vi "Untitled 3.vi"(7 "Sheet Name":string, 8 "error in":errorcluster, 9 "Value":bool, 10 "Cell Address":string, 11 "SpreadsheetDocument":refnum<k24>) -> (0 "error out":errorcluster, 3 "SpreadsheetDocument out":refnum<k24>)   [LabVIEW 2025]
uses:
  D:/git/Open-Xml-LabVIEW/dll/DocumentFormat.OpenXml.dll
  dll/DocumentFormat.OpenXml.dll
  Open Xml.lvlib
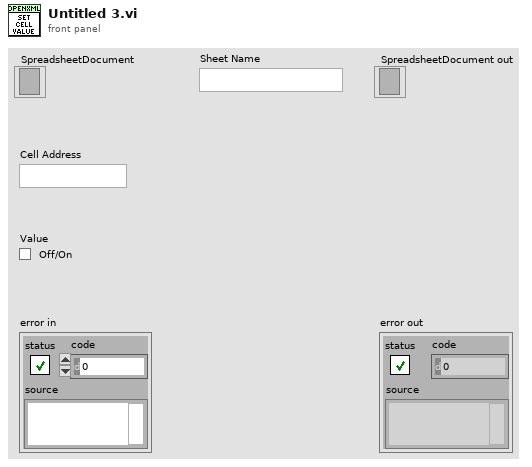
[diagram p1: front panel]
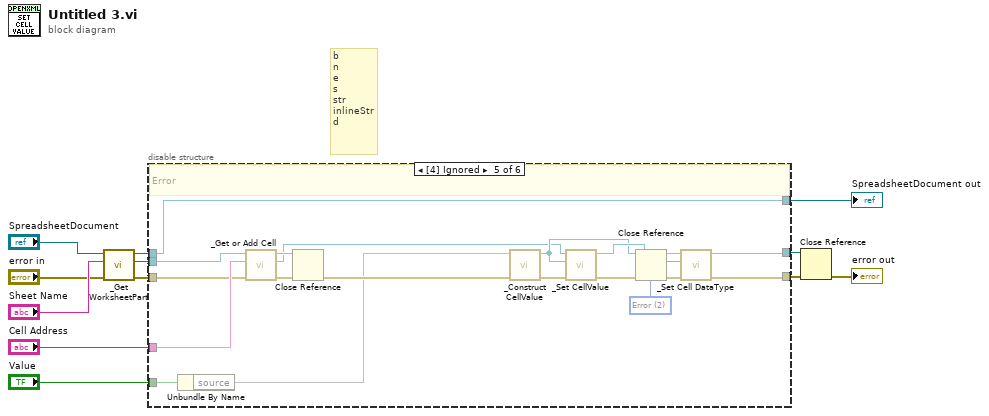
[diagram p0: block diagram]
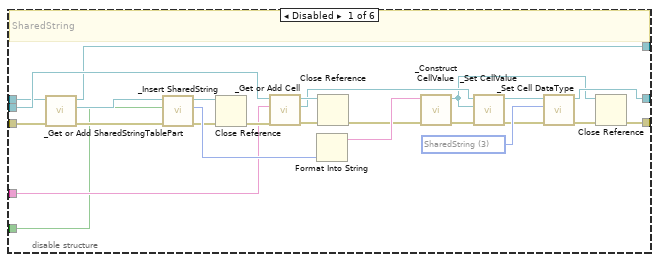
[diagram p2: hidden frame]
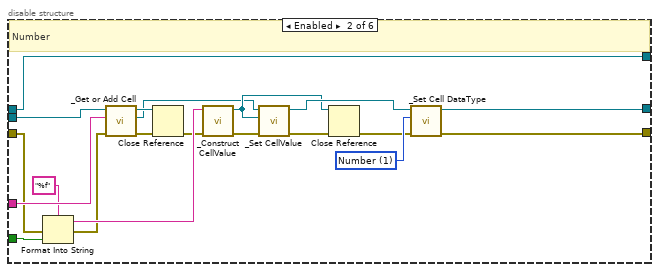
[diagram p3: hidden frame]
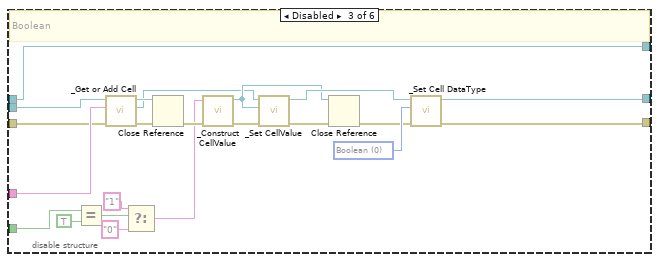
[diagram p4: hidden frame]
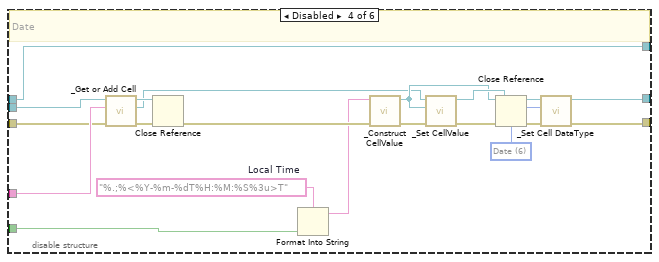
[diagram p5: hidden frame]
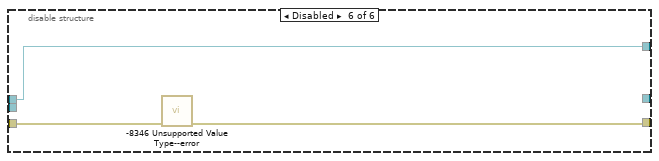
[diagram p6: hidden frame]
diagram:
  # "b\nn\ne\ns\nstr\ninlineStr\nd"
  n1 = call "_Get WorksheetPart.vi"("error in"="error in", "Sheet Name"="Sheet Name", "SpreadsheetDocument in"="SpreadsheetDocument") -> ("error out"=w8:errorcluster, "WorksheetPart"=w7:refnum<k24>, "SpreadsheetDocument out"=w3:refnum<k24>)  [unwired: 6 in]
  n2 = disable-structure shown="[4] Ignored" {
    disable-tunnel: "Value" -> [w17 w53 w64 w81 w100 _]
    disable-tunnel: "Cell Address" -> [w18 w56 w78 w97 w115 _]
    disable-tunnel: w8 -> [w37 w49 w58 w83 w101 w119]
    disable-tunnel: w7 -> [w34 w57 w79 w98 w116 _]
    disable-tunnel: [w14 w47 w74 w93 w111 w117] -> w6
    disable-tunnel: [w28 w46 w73 w92 w110 _] -> w5
    disable-tunnel: w3 -> [w20 w55 w77 w96 w114 w118]
    disable-tunnel: [w19 w55 w77 w96 w114 w118] -> w1
    frame Disabled {
      w16 = 3 items=["Boolean", "Number", "Error", "SharedString", "String", "InlineString", "Date"] ("Datatype")
      # "SharedString"
      n3 = call "_Get or Add SharedStringTablePart.vi"("error in"=w37, "SpreadsheetDoument in"=w20) -> ("error out"=w35:errorcluster, "SharedStringTablePart"=w36:refnum<k24>, "SpreadsheetDocument out"=w19:refnum<k24>)  [unwired: 7 in]
      n4 = call "_Insert SharedString.vi"("error in"=w35, "Value"=w17, "SharedStringTablePart in"=w36) -> ("error out"=w22:errorcluster, "Index"=w25:i32, "SharedStringTablePart out"=w23:refnum<k24>)  [unwired: 6 in]
      n5 = Close Reference(reference=w23, error in (no error)=w22) -> (error out=w24:errorcluster)
      n6 = call "_Get or Add Cell.vi"("error in"=w24, "Cell Address"=w18, "Worksheetpart in"=w34) -> ("error out"=w32:errorcluster, "Cell"=w21:refnum<k24>, "WorksheetPart out"=w26:refnum<k24>)  [unwired: 6 in]
      n7 = Format Into String(w25) -> (resulting string=w33:string)  [unwired: 3 in, 1 out]
      n8 = Close Reference(reference=w26, error in (no error)=w32) -> (error out=w27:errorcluster)
      n9 = call "_Construct CellValue.vi"("error in"=w27, "Text"=w33) -> ("error out"=w31:errorcluster, "CellValue out"=w13:refnum<k24>)  [unwired: 8 in]
      n10 = call "_Set CellValue.vi"("error in"=w31, "CellValue in"=w13, "Cell in"=w21) -> ("error out"=w15:errorcluster, "Cell out"=w30:refnum<k24>)  [unwired: 7 in]
      n11 = call "_Set Cell DataType.vi"("error in"=w15, "Datatype"=w16, "Cell in"=w30) -> ("error out"=w29:errorcluster, "Cell out"=w28:refnum<k24>)  [unwired: 7 in]
      n12 = Close Reference(reference=w13, error in (no error)=w29) -> (error out=w14:errorcluster)
    }
    frame Enabled {
      w43 = 1 items=["Boolean", "Number", "Error", "SharedString", "String", "InlineString", "Date"] ("Datatype")
      # "Number"
      n13 = Format Into String(format string="%f", error in=w49, w53) -> (resulting string=w51:string, error out=w48:errorcluster)  [unwired: 1 in]
      n14 = call "_Get or Add Cell.vi"("error in"=w48, "Cell Address"=w56, "Worksheetpart in"=w57) -> ("error out"=w54:errorcluster, "Cell"=w38:refnum<k24>, "WorksheetPart out"=w39:refnum<k24>)  [unwired: 6 in]
      n15 = Close Reference(reference=w39, error in (no error)=w54) -> (error out=w40:errorcluster)
      n16 = call "_Construct CellValue.vi"("error in"=w40, "Text"=w51) -> ("error out"=w50:errorcluster, "CellValue out"=w41:refnum<k24>)  [unwired: 8 in]
      n17 = call "_Set CellValue.vi"("error in"=w50, "CellValue in"=w41, "Cell in"=w38) -> ("error out"=w44:errorcluster, "Cell out"=w45:refnum<k24>)  [unwired: 7 in]
      n18 = Close Reference(reference=w41, error in (no error)=w44) -> (error out=w42:errorcluster)
      n19 = call "_Set Cell DataType.vi"("error in"=w42, "Datatype"=w43, "Cell in"=w45) -> ("error out"=w47:errorcluster, "Cell out"=w46:refnum<k24>)  [unwired: 7 in]
    }
    frame Disabled {
      w70 = 0 items=["Boolean", "Number", "Error", "SharedString", "String", "InlineString", "Date"] ("Datatype")
      # "Boolean"
      n20 = Equal?(x=w64, y=TRUE) -> (x = y?=w60:bool)
      n21 = call "_Get or Add Cell.vi"("error in"=w58, "Cell Address"=w78, "Worksheetpart in"=w79) -> ("error out"=w76:errorcluster, "Cell"=w65:refnum<k24>, "WorksheetPart out"=w66:refnum<k24>)  [unwired: 6 in]
      n22 = Select(t="1", s=w60, f="0" ("t")) -> (s? t:f=w59:string)
      n23 = Close Reference(reference=w66, error in (no error)=w76) -> (error out=w67:errorcluster)
      n24 = call "_Construct CellValue.vi"("error in"=w67, "Text"=w59) -> ("error out"=w75:errorcluster, "CellValue out"=w68:refnum<k24>)  [unwired: 8 in]
      n25 = call "_Set CellValue.vi"("error in"=w75, "CellValue in"=w68, "Cell in"=w65) -> ("error out"=w71:errorcluster, "Cell out"=w72:refnum<k24>)  [unwired: 7 in]
      n26 = Close Reference(reference=w68, error in (no error)=w71) -> (error out=w69:errorcluster)
      n27 = call "_Set Cell DataType.vi"("error in"=w69, "Datatype"=w70, "Cell in"=w72) -> ("error out"=w74:errorcluster, "Cell out"=w73:refnum<k24>)  [unwired: 7 in]
    }
    frame Disabled {
      w82 = "%.;%<%Y-%m-%dT%H:%M:%S%3u>T"  # Local Time
      w89 = 6 items=["Boolean", "Number", "Error", "SharedString", "String", "InlineString", "Date"] ("Datatype")
      # "Date"
      n28 = call "_Get or Add Cell.vi"("error in"=w83, "Cell Address"=w97, "Worksheetpart in"=w98) -> ("error out"=w95:errorcluster, "Cell"=w84:refnum<k24>, "WorksheetPart out"=w85:refnum<k24>)  [unwired: 6 in]
      n29 = Close Reference(reference=w85, error in (no error)=w95) -> (error out=w86:errorcluster)
      n30 = Format Into String(format string=w82, w81) -> (resulting string=w80:string)  [unwired: 2 in, 1 out]
      n31 = call "_Construct CellValue.vi"("error in"=w86, "Text"=w80) -> ("error out"=w94:errorcluster, "CellValue out"=w87:refnum<k24>)  [unwired: 8 in]
      n32 = call "_Set CellValue.vi"("error in"=w94, "CellValue in"=w87, "Cell in"=w84) -> ("error out"=w90:errorcluster, "Cell out"=w91:refnum<k24>)  [unwired: 7 in]
      n33 = Close Reference(reference=w87, error in (no error)=w90) -> (error out=w88:errorcluster)
      n34 = call "_Set Cell DataType.vi"("error in"=w88, "Datatype"=w89, "Cell in"=w91) -> ("error out"=w93:errorcluster, "Cell out"=w92:refnum<k24>)  [unwired: 7 in]
    }
    frame Disabled {
      w107 = 2 items=["Boolean", "Number", "Error", "SharedString", "String", "InlineString", "Date"] ("Datatype")
      # "Error"
      n35 = Unbundle By Name(w100) -> ("source"=w99)
      n36 = call "_Get or Add Cell.vi"("error in"=w101, "Cell Address"=w115, "Worksheetpart in"=w116) -> ("error out"=w113:errorcluster, "Cell"=w102:refnum<k24>, "WorksheetPart out"=w103:refnum<k24>)  [unwired: 6 in]
      n37 = Close Reference(reference=w103, error in (no error)=w113) -> (error out=w104:errorcluster)
      n38 = call "_Construct CellValue.vi"("error in"=w104, "Text"=w99) -> ("error out"=w112:errorcluster, "CellValue out"=w105:refnum<k24>)  [unwired: 8 in]
      n39 = call "_Set CellValue.vi"("error in"=w112, "CellValue in"=w105, "Cell in"=w102) -> ("error out"=w108:errorcluster, "Cell out"=w109:refnum<k24>)  [unwired: 7 in]
      n40 = Close Reference(reference=w105, error in (no error)=w108) -> (error out=w106:errorcluster)
      n41 = call "_Set Cell DataType.vi"("error in"=w106, "Datatype"=w107, "Cell in"=w109) -> ("error out"=w111:errorcluster, "Cell out"=w110:refnum<k24>)  [unwired: 7 in]
    }
    frame Disabled {
      n42 = call "-8346 Unsupported Value Type--error.vi"("error in"=w119) -> ("error out"=w117:errorcluster)  [unwired: 10 in]
    }
  }
  "SpreadsheetDocument out" <- w1
  n43 = Close Reference(reference=w5, error in (no error)=w6) -> (error out=→"error out":errorcluster)
